vi "uTransport_Event_Create.vi"(8 "error in (no error)":errorcluster) -> (0 "error out":errorcluster, 2 "Event:uMsg":refnum<event-registration>, 3 "uTransport_Event out":refnum<class "uTransport_Event.lvclass">)   [LabVIEW 2023, in "uLib.lvlib" / "uTransport_Event.lvclass"]
doc: "Do not destroy the event except after the listener loop has stopped."
uses:
  uTransport_Event.lvclass
  uMsg/uMsg/uMsg.lvclass
  uTransport_Event.lvclass/uTransport_Event.ctl
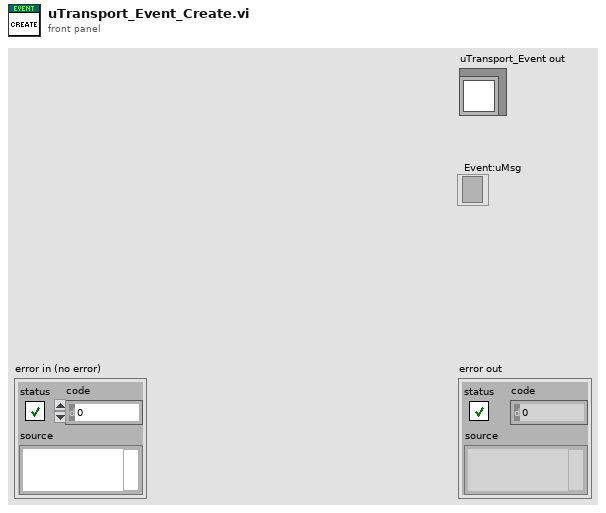
[diagram p1: front panel]
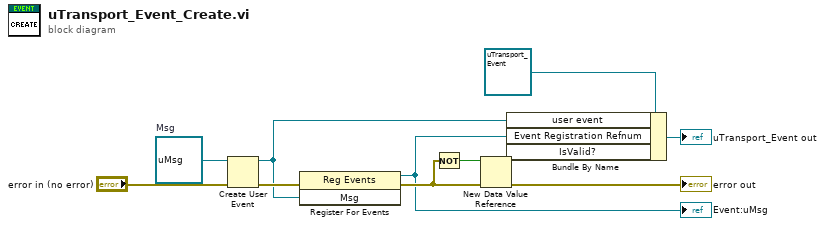
[diagram p0: block diagram]
diagram:
  w7 = refnum<class "uMsg.lvclass"> refnum  # Msg
  n1 = Create User Event(user event datatype=w7, error in="error in (no error)") -> (user event=w4:refnum<user-event>, error out=w6:errorcluster)
  n2 = register-events(error in=w6, w4) -> (reference out=w3:refnum<event-registration>, error out=w11:errorcluster)  [unwired: 1 in]
  "Event:uMsg" <- w3
  n3 = Not(x=w11) -> (.not. x?=w2:bool)
  n4 = New Data Value Reference(data value=w2, error in=w11) -> (data value reference=w1:refnum<data-value>, error out=→"error out":errorcluster)
  n5 = Bundle By Name(cluster=refnum<class "uTransport_Event.lvclass"> refnum ("uTransport_Event out"), "user event"=w4, "Event Registration Refnum"=w3, "IsValid?"=w1) -> (→"uTransport_Event out":refnum<class "uTransport_Event.lvclass">)
